vi "2_PixelToMicronConversion (SubVI).vi"(8 "error in (no error)":errorcluster, 9 "Template Image":path=path "C:/Users/Aerotech/Documents/BNL_ThermomechanicalStave/0_Calibration/1_Camera/2_10Strips_PixMicronCalibTemplate_10mpx_4_20.png", 11 "Images Array":T1[](array[plugin-control])=["image_000_-650_100_-22"]) -> (0 "error out":errorcluster, 1 "Average microns/pixel":ext=1.578484391246922, 3 "standard dev on microns/pixel":ext=nan)   [LabVIEW 2016]
doc: "This example shows how to use the geometric matching tools in NI Vision.\n\nGeometric matching is the technique used to quickly locate known reference or fiducial patterns in an image using edge information. Geometric matching is the key to many applications. Geometric matching can provide your application with information about the presence or absence, number, and location of the model within an image.\n\nAn important step in geometric matching is training the template. A specialized geometric training interface is provided for simple training with advanced features. This utility can be found at Start»Programs»National Instruments»Vision, or from Vision Assistant or Vision Builder for Automated Inspection."
uses:
  <vilib>/vision/Pattern Matching.llb/IMAQ Match Range Setting.ctl
  <vilib>/vision/NI_Vision_Development_Module.lvlib
  <vilib>/Analysis/NI_AALBase.lvlib
panel:
  in  "Testing?":bool
  in  "Images Directory":path=path "C:/Users/Aerotech/cernbox/BNL/Stave Assembly Records/2017-04-18/pix_um_calib"
  in  "Naming Convention":string="*.png"
  in  "Range Settings":T2[](array[typedef])=[{"Match Constraints"=1, "Min"=75.0, "Max"=125.0}] {"Max" format="%.2f"; "Min" format="%.2f"; "Match Constraints" items=["Rotation Angle (degrees)", "Scale Factor (%)", "Occlusion (%)"]}
  out "Results":string[][](table)=[["0"], ["2296.60"], ["1609.01"], ["358.21"], ["100.06"], ["998.94"], ["0.00"], ["998.94"], ["0.00"], ["999.57"]]
  in  "Minimum Score":sgl=800.0
  in  "Number of Matches":i32=1
  out "Template":T1(plugin-control)
  out "Image":T1(plugin-control)
  # "Overview: This takes a set of images which include strips and a template (given) and finds the pixel to micron ratio average and standard deviation across images. \nRequirements: NI Vision Development Module\nInstructions: Select an image in your path and naming convention of images.  Run to find microns/pixel and standard deviation.\n\nBUILT BY LAURA BERGSTEN FROM THE \"Geometric Matching.vi\" example from NI"
  # "Range"
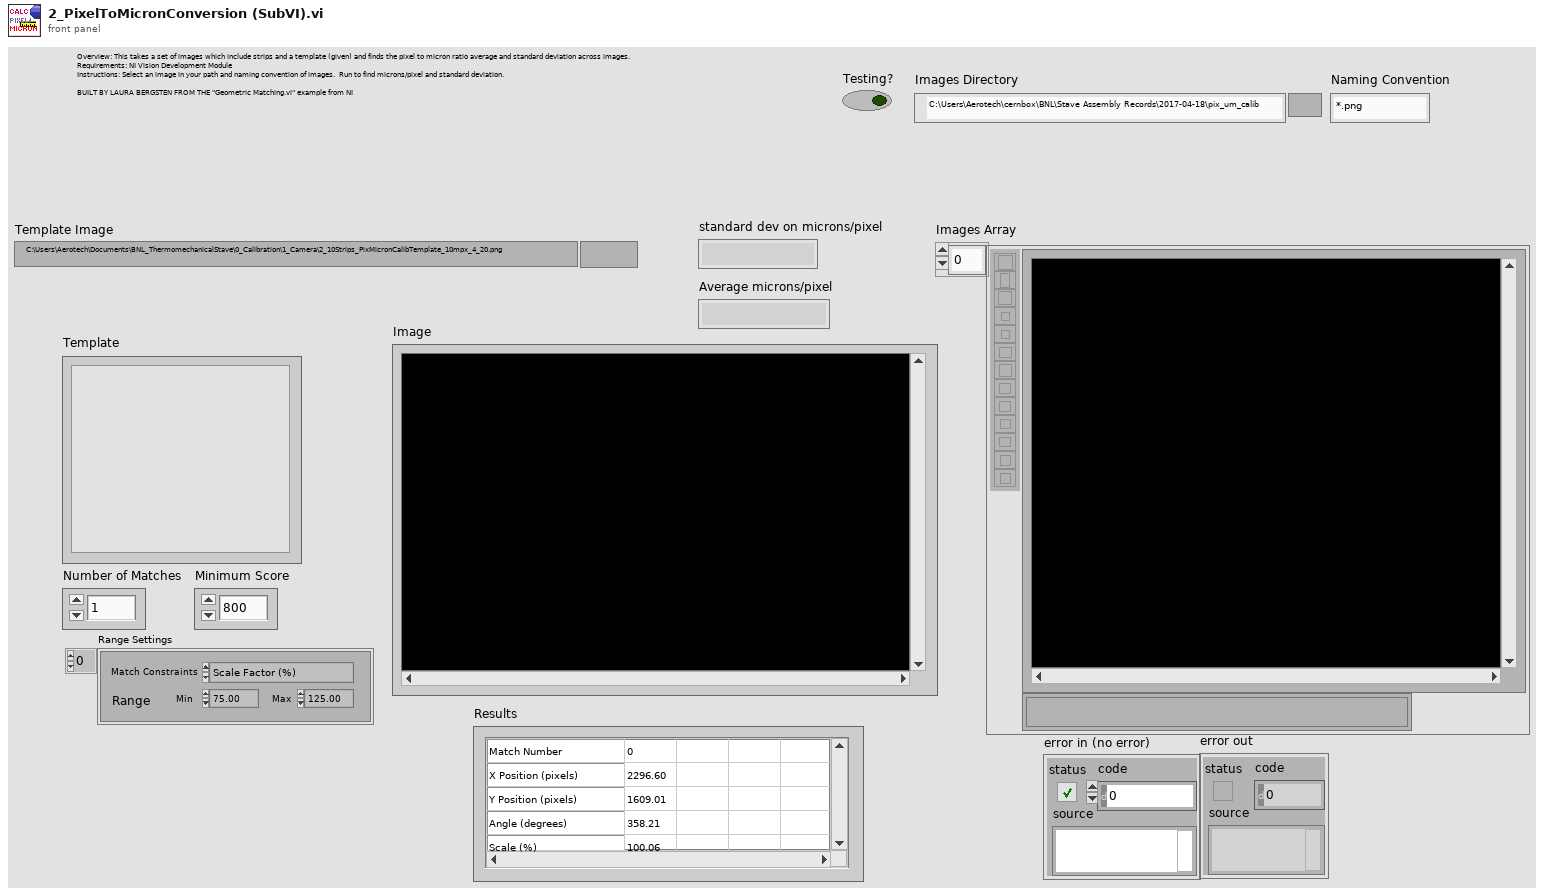
[diagram p1: front panel]
types:
  T1 = typedef "IMAQ Image.ctl" = refnum<image>
  T2 = typedef "IMAQ Match Range Setting.ctl" = cluster{"Match Constraints":u32, "Min":dbl, "Max":dbl}
  T3 = typedef "Image Type" = u32
  T4 = cluster{"Rotation":bool, "Scale":bool, "Occlusion":bool, "Reserved":bool, "Reserved":bool, "Reserved":bool}
  T5 = typedef "IMAQ GM Match Report.ctl" = cluster{"Position":cluster{"x":sgl, "y":sgl}, "Angle":sgl, "Scale":sgl, "Score":sgl, "Bounding Box":cluster{"x":sgl, "y":sgl}[], "Contrast Reversed":bool, "Occlusion %":sgl, "Template Target Curve Score":sgl, "Target Template Curve Score":sgl, "Correlation Score":sgl}
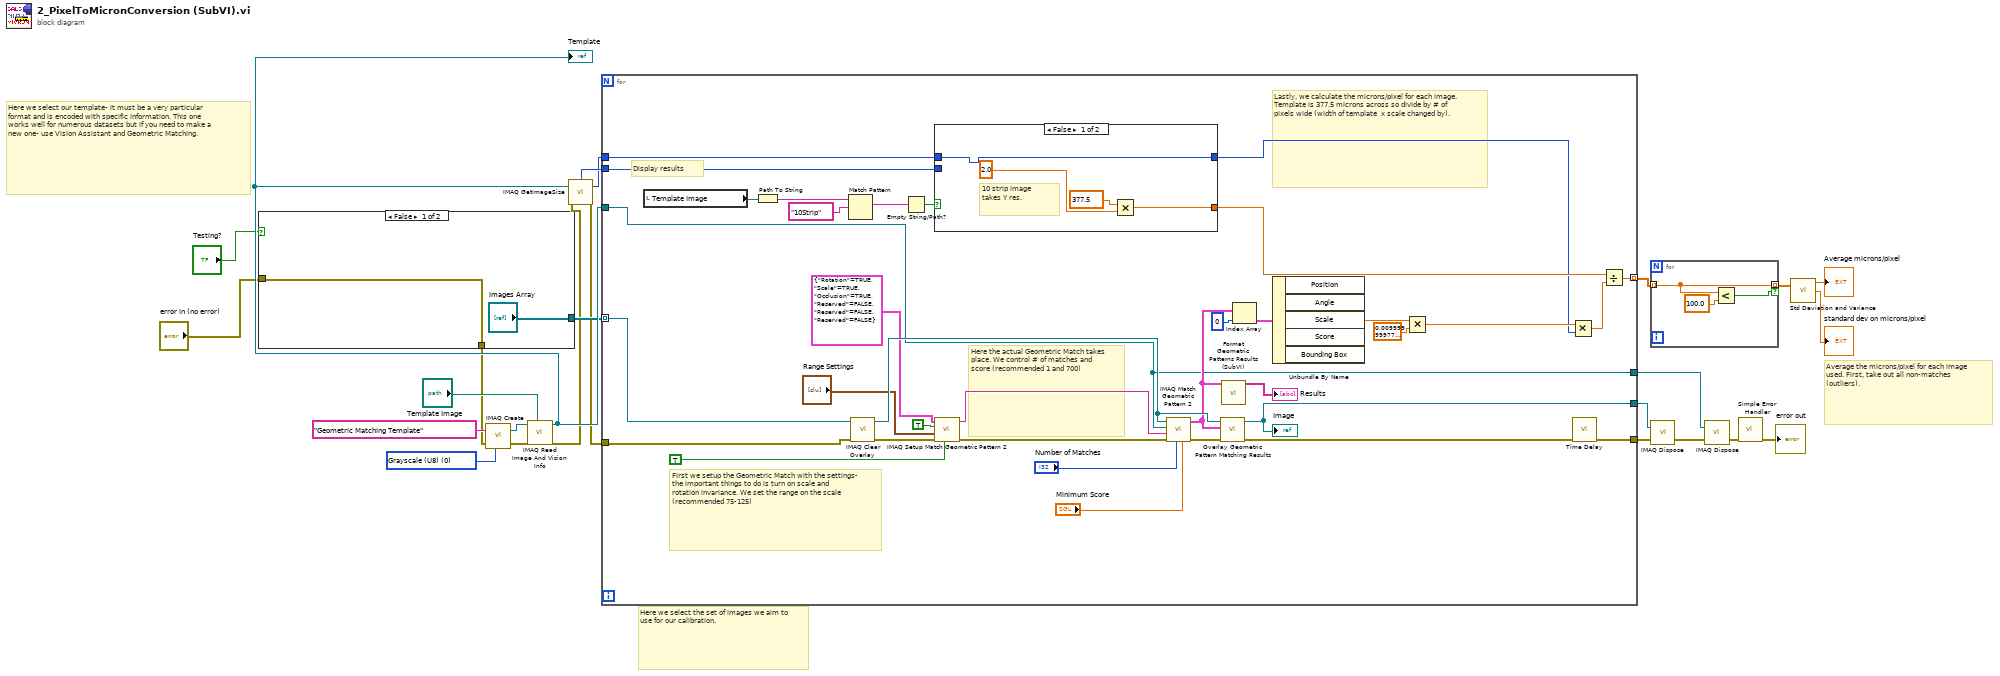
[diagram p0: block diagram]
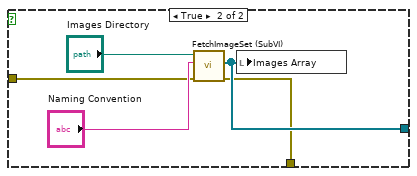
[diagram p2: hidden frame]
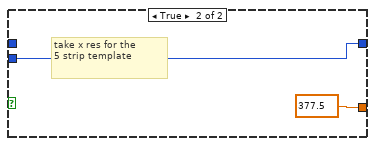
[diagram p3: hidden frame]
diagram:
  w21 = T3 0 items=["Grayscale (U8)", "Grayscale (I16)", "Grayscale (SGL)", "Complex (CSG)", "RGB (U32)", "HSL (U32)", "RGB (U64)"] ("Image Type")
  # "Average the microns/pixel for each image used. First, take out all non-matches (outliers)."
  # "Here we select the set of images we aim to use for our calibration."
  # "Here we select our template- it must be a very particular format and is encoded with specific information. This one works well for numerous datasets but if you need to make a new one- use Vision Assistant and Geometric Matching."
  n1 = case shown="False" "Testing?" {
    tunnel: ["Images Array" w29] -> w8
    tunnel: "error in (no error)" -> [w25 w28]
    tunnel: [w25 w27] -> w4
    frame False {
    }
    frame True {
      n2 = call "FetchImageSet (SubVI).vi"("error in (no error)"=w28, "Naming Convention"="Naming Convention", "Images Directory"="Images Directory") -> ("error out"=w27:errorcluster, "Image Array"=w29:T1[])  [unwired: 6 in, 1 out]
      n3 = local write "Images Array"(w29) -> ()
    }
  }
  n4 = call "IMAQ Create"("Image Name"="Geometric Matching Template", "Image Type"=w21, "error in (no error)"=w4) -> ("New Image"=w22:T1, "error out"=w23:errorcluster)  [unwired: 1 in, 1 out]
  n5 = call "IMAQ Read Image And Vision Info"("File Path"="Template Image", "error in (no error)"=w23, "Image"=w22) -> ("error out"=w3:errorcluster, "Image Out"=w15:T1)  [unwired: 1 in, 6 out]
  "Template" <- w15
  n6 = call "IMAQ GetImageSize"("Image"=w15, "error in (no error)"=w3) -> ("Y Resolution"=w7:i32, "X Resolution"=w14:i32, "error out"=w2:errorcluster)  [unwired: 2 in]
  n7 = for {
    tunnel: [w66] -> w24
    tunnel: w15 -> [w32]
    tunnel: [w42] -> w19
    tunnel: w2 -> [w44]
    tunnel: [w49] -> w10 mode=indexing
    tunnel: w14 -> [w35]
    tunnel: w8 -> [w43] mode=indexing
    tunnel: w7 -> [w33]
    tunnel: [w32] -> w6
    # "Display results"
    # "Here the actual Geometric Match takes place. We control # of matches and score (recommended 1 and 700)"
    # "First we setup the Geometric Match with the settings- the important things to do is turn on scale and rotation invariance. We set the range on the scale (recommended 75-125)"
    # "Lastly, we calculate the microns/pixel for each image. Template is 377.5 microns across so divide by # of pixels wide (width of template  x scale changed by)."
    n8 = local read "Template Image"() -> (w41:path)
    n9 = Path To String(path=w41) -> (string=w40:string)
    n10 = Match Pattern(string=w40, regular expression="10Strip") -> (match substring=w38:string)  [unwired: 1 in, 3 out]
    n11 = call "IMAQ Clear Overlay"("error in (no error)"=w44, "Image"=w43) -> ("error out"=w60:errorcluster, "Image Out"=w58:T1)  [unwired: 1 in, 7 out]
    n12 = Empty String/Path?(string/path=w38) -> (empty?=w37:bool)
    n13 = case shown="False" w37 {
      tunnel: [w69 377.5 ("x")] -> w36
      tunnel: [w67 w71] -> w34
      tunnel: w35 -> [_ w71]
      tunnel: w33 -> [w67 _]
      frame False {
        # "10 strip image\ntakes Y res."
        n14 = Multiply(x=377.5, y=2.0) -> (x*y=w69:dbl)
      }
      frame True {
        # "take x res for the\n5 strip template"
      }
    }
    n15 = call "IMAQ Setup Match Geometric Pattern 2"("Use Learn Curve Parameters"=TRUE, "error in (no error)"=w60, "Range Settings"="Range Settings", "Subpixel Accuracy"=TRUE, "Match Mode"=T4 {"Rotation"=TRUE, "Scale"=TRUE, "Occlusion"=TRUE, "Reserved"=FALSE, "Reserved"=FALSE, "Reserved"=FALSE}) -> ("error out"=w65:errorcluster, "Match Geometric Pattern 2 Setup Data"=w45:string)  [unwired: 1 in, 4 out]
    n16 = call "IMAQ Match Geometric Pattern 2"("Minimum Match Score"="Minimum Score", "Number of Matches Requested"="Number of Matches", "error in (no error)"=w65, "Match Geometric Pattern 2 Setup Data"=w45, "Template Image"=w32, "Image"=w58) -> ("error out"=w61:errorcluster, "Matches (pixel)"=w56:T5[])  [unwired: 1 in, 3 out]
    n17 = call "Overlay Geometric Pattern Matching Results.vi"("error in"=w61, "Matches"=w56, "Image"=w58) -> ("error out"=w59:errorcluster, "Image Out"=w42:T1)  [unwired: 2 in, 5 out]
    "Image" <- w42
    n18 = call "Format Geometric Patterns Results (SubVI).vi"("Matches"=w56) -> ("Text Results"=→"Results":string[][])  [unwired: 9 in, 1 out]
    n19 = Index Array(array=w56, index=0) -> (element=w54:T5)
    n20 = Unbundle By Name(w54) -> ("Scale"=w53:sgl)  [unwired: 4 out]
    n21 = Multiply(x=w53, y=sgl 0.01) -> (x*y=w51:sgl)
    n22 = Multiply(x=w51, y=w34) -> (x*y=w50:sgl)
    n23 = call "Time Delay"("error in (no error)"=w59) -> ("error out"=w66:errorcluster)  [unwired: 10 in]
    n24 = Divide(x=w36, y=w50) -> (x/y=w49:dbl)
  }
  n25 = for {
    tunnel: w10 -> [w74] mode=indexing
    tunnel: [w74] -> w11 mode=indexing if=w73
    n26 = Less?(x=w74, y=100.0) -> (x < y?=w73:bool)
  }
  n27 = call "IMAQ Dispose"("Image"=w19, "error in (no error)"=w24) -> ("error out"=w18:errorcluster)  [unwired: 1 in, 3 out]
  n28 = call "IMAQ Dispose"("Image"=w6, "error in (no error)"=w18) -> ("error out"=w17:errorcluster)  [unwired: 1 in, 3 out]
  n29 = call <vilib>:"Simple Error Handler.vi"("error in (no error)"=w17) -> ("error out"=→"error out":errorcluster)  [unwired: 4 in, 4 out]
  n30 = call <vilib>:"Std Deviation and Variance.vi"("X"=w11) -> ("mean"=→"Average microns/pixel":dbl, "standard deviation"=→"standard dev on microns/pixel":dbl)  [unwired: 1 in, 1 out]
